vi "AE_threshold_wPlot.vi"() -> ()   [LabVIEW 2012]
uses:
  <vilib>/DAQmx/read.llb/DAQmx Read (Analog 1D Wfm NChan NSamp).vi
  <vilib>/DAQmx/create/channels.llb/DAQmx Create Channel (AI-Voltage-Basic).vi
  <vilib>/DAQmx/configure/timing.llb/DAQmx Timing (Sample Clock).vi
  <vilib>/DAQmx/miscellaneous.llb/DAQmx Fill In Error Info.vi
panel:
  out "Wavelets":waveform(dbl)[](graph)
  in  "Threshold Method":u16(ring) items=["Max", "Amplitude", "Rising Value"]
  in  "Threshold (V)":dbl=0.01 min=0.0 max=10.0 step=0.001 format="%0.3f"
  in  "Physical Channel":tag="Dev1/ai7"
  in  "Gain":u16(ring)=1 items=["20 dB", "40 dB", "60 dB"]
  out "Events":i32
  in  "Sample Window (us)":i32=500 min=0 max=1000
  in  "stop":bool
  in  "Test Name":string="test"
  in  "Storage Directory":path=path "C:/Users/User/Desktop/Users_2013-2014/Michael Rossol"
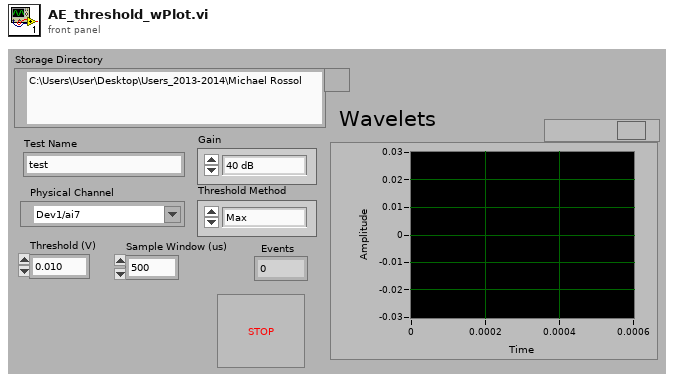
[diagram p1: front panel]
types:
  T1 = enum16{"open", "open or create", "create or replace", "create", "open (read only)"}
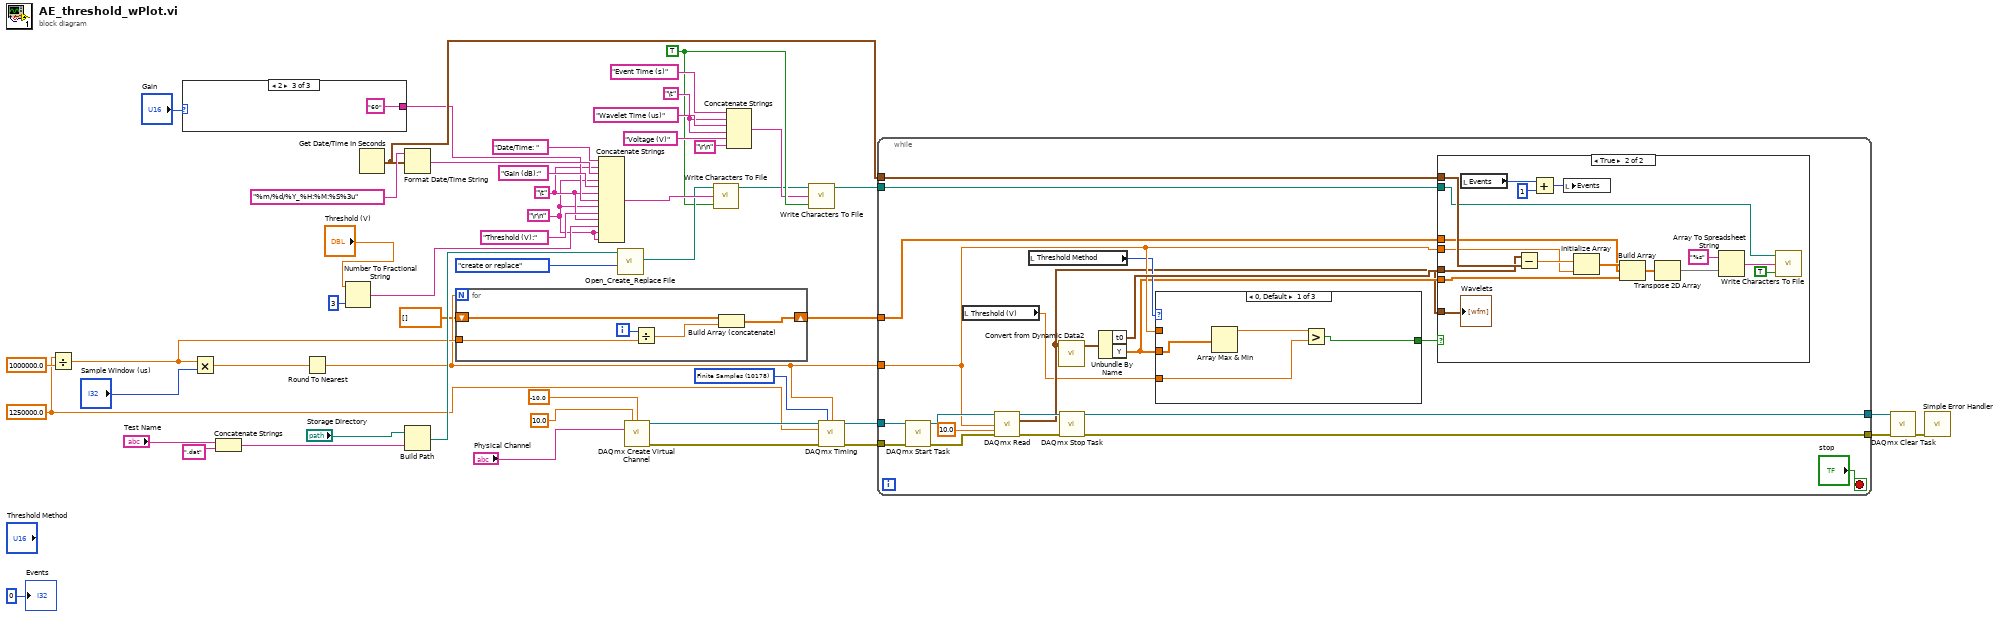
[diagram p0: block diagram]
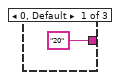
[diagram p2: hidden frame]
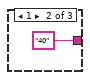
[diagram p3: hidden frame]
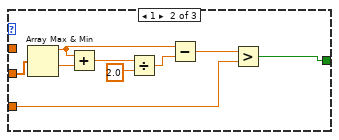
[diagram p4: hidden frame]
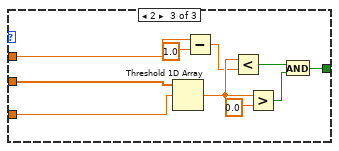
[diagram p5: hidden frame]
diagram:
  w18 = 10178 items=["Finite Samples"=10178, "Continuous Samples"=10123] ("sample mode")
  w32 = "\t"
  w17 = 1250000.0 ("x")
  w5 = "\t"
  w1 = "\r\n"
  w29 = TRUE ("append to file? (new file:F)")
  n1 = Divide(x=w17, y=1000000.0) -> (x/y=w35:dbl)
  n2 = case shown="2" "Gain" {
    tunnel: ["20" ("string") "40" ("string") "60" ("string")] -> w23
    frame 0, Default {
    }
    frame 1 {
    }
    frame 2 {
    }
  }
  n3 = Multiply(x=w35, y="Sample Window (us)") -> (x*y=w11:dbl)
  n4 = Concatenate Strings("Test Name", ".dat" ("string")) -> (w43:string)
  n5 = Round To Nearest(number=w11) -> (nearest integer value=w10:dbl)
  n6 = Number To Fractional String(number="Threshold (V)", precision (6)=i16 3) -> (F-format string=w3:string)  [unwired: 2 in]
  n7 = Get Date/Time In Seconds() -> (seconds since 1Jan1904=w36:timestamp)
  n8 = Format Date/Time String(time format string (%c)="%m/%d/%Y_%H:%M:%S%3u", seconds (now)=w36) -> (date/time string=w40:string)  [unwired: 1 in]
  n9 = Build Path(base path="Storage Directory", name or relative path=w43) -> (appended path=w41:path)
  n10 = for {
    N: w10 -> [_]
    shift-right: [w57] -> w9
    shift-left: dbl[] [] -> [w58]
    tunnel: w35 -> [w54]
    i -> [w56]
    n11 = Divide(x=w56, y=w54) -> (x/y=w55:dbl)
    n12 = Build Array (concatenate)(w58, w55) -> (w57:dbl[])
  }
  n13 = Concatenate Strings("Date/Time: ", w5, w40, w1, "Gain (dB):" ("string"), w5, w23, w1, "Threshold (V):" ("string"), w5, w3, w1, w1) -> (w50:string)
  n14 = call <vilib>:"Open_Create_Replace File.vi"("function (open:0)"=T1."create or replace", "file path"=w41) -> ("new file path"=w46:path)  [unwired: 6 in, 3 out]
  n15 = call-poly <vilib>:"DAQmx Create Virtual Channel.vi"("maximum value"=10.0, "minimum value"=-10.0, "physical channels"="Physical Channel") -> ("task out"=w20:refnum<k21>, "error out"=w19:errorcluster)  [unwired: 11 in]
  n16 = call <vilib>:"Write Characters To File.vi"("append to file? (new file:F)"=w29, "character string"=w50, "file path (dialog if empty)"=w46) -> ("new file path (Not A Path if cancelled)"=w27:path)  [unwired: 2 in]
  n17 = Concatenate Strings("Event Time (s)" ("string"), w32, "Wavelet Time (us)" ("string"), w32, "Voltage (V)" ("string"), "\r\n") -> (w28:string)
  n18 = call <vilib>:"Write Characters To File.vi"("append to file? (new file:F)"=w29, "character string"=w28, "file path (dialog if empty)"=w27) -> ("new file path (Not A Path if cancelled)"=w26:path)  [unwired: 2 in]
  n19 = call-poly <vilib>:"DAQmx Timing.vi"("task/channels in"=w20, "sample mode"=w18, "samples per channel"=w10, "rate"=w17, "error in"=w19) -> ("task out"=w16:refnum<k21>, "error out"=w15:errorcluster)  [unwired: 9 in]
  n20 = while {
    tunnel: w26 -> [w68]
    tunnel: w10 -> [w63]
    tunnel: w36 -> [w69]
    tunnel: w9 -> [w65]
    tunnel: w16 -> [w71]
    tunnel: w15 -> [w70]
    tunnel: [w73] -> w13
    tunnel: [w72] -> w12
    stop <- "stop" stop-if-true
    n21 = call <vilib>:"DAQmx Start Task.vi"("task/channels in"=w71, "error in"=w70) -> ("task out"=w78:refnum<k21>, "error out"=w77:errorcluster)  [unwired: 12 in]
    n22 = local read "Threshold (V)"() -> (w59:dbl)
    n23 = call-poly <vilib>:"DAQmx Read.vi"("task/channels in"=w78, "number of samples per channel"=w63, "timeout"=10.0, "error in"=w77) -> ("task out"=w74:refnum<k21>, "data"=w60:waveform(dbl)[], "error out"=w75:errorcluster)  [unwired: 9 in]
    n24 = local read "Threshold Method"() -> (w62:u16)
    n25 = call "Convert from Dynamic Data2"("Dynamic Data Type"=w60) -> ("Waveform"=w67:waveform(dbl))  [unwired: 3 in]
    n26 = call <vilib>:"DAQmx Stop Task.vi"("task/channels in"=w74, "error in"=w75) -> ("task out"=w72:refnum<k21>, "error out"=w73:errorcluster)  [unwired: 12 in]
    n27 = Unbundle By Name(w67) -> ("t0"=w66:timestamp, "Y"=w61:dbl[])
    n28 = case shown="0, Default" w62 {
      tunnel: w61 -> [w80 w84 w100]
      tunnel: [w82 w86 w96] -> w64
      tunnel: w63 -> [_ _ w95]
      tunnel: w59 -> [w81 w85 w93]
      frame 0, Default {
        n29 = Array Max & Min(array=w80) -> (max value=w83:dbl)  [unwired: 3 out]
        n30 = Greater?(x=w83, y=w81) -> (0:w82:bool)
      }
      frame 1 {
        n31 = Array Max & Min(array=w84) -> (max value=w88:dbl, min value=w92:dbl)  [unwired: 2 out]
        n32 = Add(x=w88, y=w92) -> (x+y=w91:dbl)
        n33 = Divide(x=w91, y=2.0) -> (x/y=w89:dbl)
        n34 = Subtract(x=w88, y=w89) -> (x-y=w87:dbl)
        n35 = Greater?(x=w87, y=w85) -> (0:w86:bool)
      }
      frame 2 {
        n36 = Threshold 1D Array(2:w93, 3:w100) -> (0:w101:dbl)  [unwired: 1 in]
        n37 = Subtract(x=w95, y=1.0) -> (x-y=w99:dbl)
        n38 = Less?(x=w101, y=w99) -> (x < y?=w98:bool)
        n39 = Greater?(x=w101, y=0.0) -> (0:w97:bool)
        n40 = And(x=w98, y=w97) -> (x .and. y?=w96:bool)
      }
    }
    n41 = case shown="True" w64 {
      tunnel: w69 -> [_ w112]
      tunnel: w63 -> [_ w111]
      tunnel: w68 -> [_ w110]
      tunnel: w66 -> [_ w109]
      tunnel: w65 -> [_ w108]
      tunnel: w61 -> [_ w107]
      tunnel: w60 -> [_ w103]
      frame False {
      }
      frame True {
        n42 = local read "Events"() -> (w104:i32)
        n43 = Subtract(x=w109, y=w112) -> (x-y=w116:dbl)
        n44 = Add(x=w104, y=1) -> (x+y=w105:i32)
        n45 = local write "Events"(w105) -> ()
        n46 = Initialize Array(w116, w111) -> (w115:dbl[])
        n47 = Build Array(w115, w108, w107) -> (w114:dbl[][])
        n48 = Transpose 2D Array(2D array=w114) -> (transposed array=w113:dbl[][])
        n49 = Array To Spreadsheet String(array=w113, 3:"%s" ("format string")) -> (spreadsheet string=w118:string)  [unwired: 1 in]
        n50 = call <vilib>:"Write Characters To File.vi"("append to file? (new file:F)"=TRUE, "character string"=w118, "file path (dialog if empty)"=w110) -> ()  [unwired: 2 in, 1 out]
        "Wavelets" <- w103
      }
    }
  }
  n51 = call <vilib>:"DAQmx Clear Task.vi"("task in"=w12, "error in"=w13) -> ("error out"=w14:errorcluster)  [unwired: 13 in]
  n52 = call <vilib>:"Simple Error Handler.vi"("error in (no error)"=w14) -> ()  [unwired: 4 in, 5 out]
  "Events" <- 0
